vi "Push and hold.vi"(3 "Reset":bool, 4 "Input":bool) -> (1 "Output":bool)   [LabVIEW 2019]
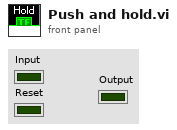
[diagram p1: front panel]
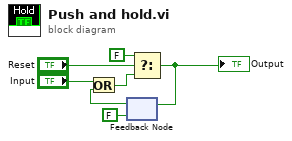
[diagram p0: block diagram]
diagram:
  n1 = feedback #1(FALSE) -> (w6:bool)
  n2 = Or(x="Input", y=w6) -> (x .or. y?=w4:bool)
  n3 = Select(t=FALSE, s="Reset", f=w4) -> (s? t:f=w1:bool)
  "Output" <- w1
  n4 = feedback-in #1(w1) -> ()
